vi "Configure OCP.vi"(6 "Protection Delay (0)":dbl min=0.0 max=60.0 step=1.0 format="%#.0g", 8 "error in (no error)":errorcluster, 9 "Enable OCP (T: Enable)":bool=TRUE, 10 "Current Limit (15.000 A)":dbl=15.0 min=0.0 max=240.0 step=0.001 format="%.3g", 11 "VISA resource name":refnum<visa-resource-name>) -> (0 "error out":errorcluster, 3 "VISA resource name out":refnum<visa-resource-name>)   [LabVIEW 2018, in "BK Precision 8600 Series.lvlib"]
doc: "Configures over current protection (OCP). Specify the current limit, protection delay, and whether to enable or disable OCP."
uses:
  <instrlib>/BK Precision 8600 Series/BK Precision 8600 Series.lvlib
panel:
  # "s"
  # "A"
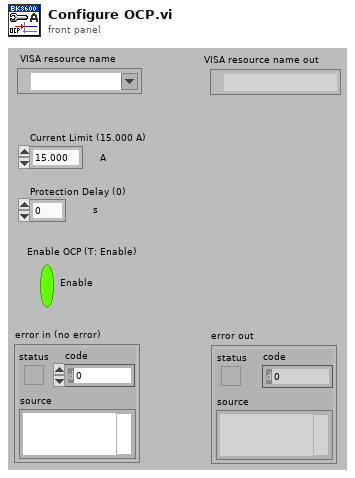
[diagram p1: front panel]
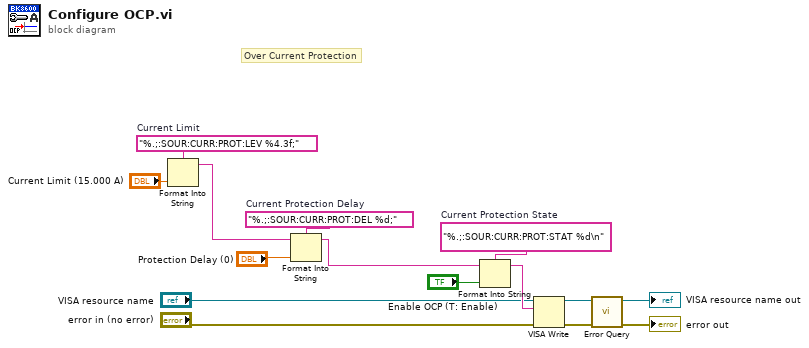
[diagram p0: block diagram]
diagram:
  w12 = "%.;:SOUR:CURR:PROT:DEL %d;"  # Current Protection Delay
  w13 = "%.;:SOUR:CURR:PROT:STAT %d\n"  # Current Protection State
  w15 = "%.;:SOUR:CURR:PROT:LEV %4.3f;"  # Current Limit
  # "Over Current Protection"
  n1 = Format Into String(format string=w15, "Current Limit (15.000 A)") -> (resulting string=w11:string)  [unwired: 2 in, 1 out]
  n2 = Format Into String(format string=w12, initial string=w11, "Protection Delay (0)") -> (resulting string=w10:string)  [unwired: 1 in, 1 out]
  n3 = Format Into String(format string=w13, initial string=w10, "Enable OCP (T: Enable)") -> (resulting string=w14:string)  [unwired: 1 in, 1 out]
  n4 = VISA Write(VISA resource name="VISA resource name", write buffer=w14, error in (no error)="error in (no error)") -> (VISA resource name out=w6:refnum<visa-resource-name>, error out=w5:errorcluster)  [unwired: 1 out]
  n5 = call <instrlib>:"Error Query.vi"("error in (no error)"=w5, "VISA resource name"=w6) -> ("error out"=→"error out":errorcluster, "VISA resource name out"=→"VISA resource name out":refnum<visa-resource-name>)  [unwired: 6 in, 2 out]
